vi "Destory User Que.vi"(8 "error in":errorcluster, 11 "queVariant":refnum<queue>) -> (0 "error out":errorcluster)   [LabVIEW 2016]
uses:
  Event/Ctl/EventVariantData.ctl
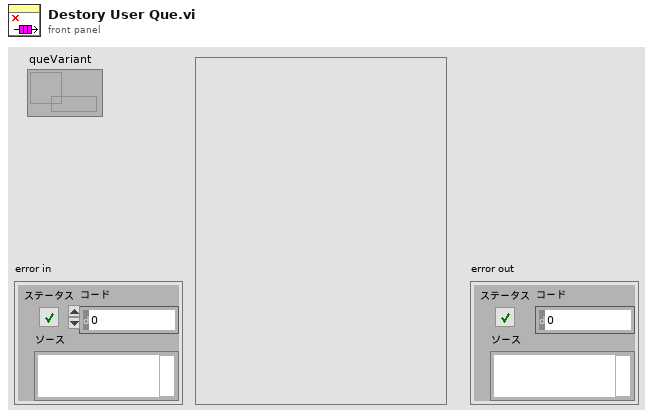
[diagram p1: front panel]
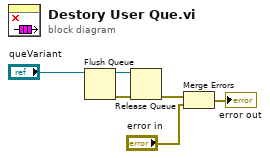
[diagram p0: block diagram]
diagram:
  n1 = Flush Queue(queue="queVariant") -> (queue out=w5:refnum<queue>, error out=w6:errorcluster)  [unwired: 1 in, 1 out]
  n2 = Release Queue(queue=w5, error in (no error)=w6) -> (error out=w3:errorcluster)  [unwired: 1 in, 2 out]
  n3 = Merge Errors(w3, "error in") -> (→"error out":errorcluster)
